vi "Set Frame Position (Time).vi"(8 "error in (no error)":errorcluster, 10 "Time (ms)":u64, 11 "Reader in":refnum<class "Reader.lvclass">) -> (0 "error out":errorcluster, 3 "Reader":refnum<class "Reader.lvclass">)   [LabVIEW 2020, in "video_io.lvlib" / "Reader.lvclass"]
uses:
  Reader.lvclass
  Reader.lvclass/Reader.ctl
  acb2feee-aaa4-4f40-955f-c8ac8e9dff35.vi
  <vilib>/Utility/error.llb/Error Cluster From Error Code.vi
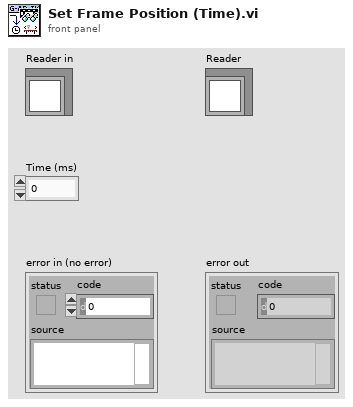
[diagram p1: front panel]
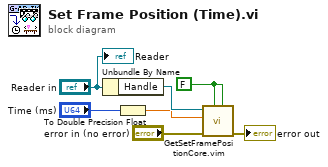
[diagram p0: block diagram]
diagram:
  w1 = FALSE ("Get")
  n1 = Unbundle By Name("Reader in") -> ("Handle"=w7:refnum<data-value>)
  n2 = To Double Precision Float(number="Time (ms)") -> (double precision float=w3:dbl)
  n3 = call "GetSetFramePositionCore.vim"("As Frame Index"=w1, "Get"=w1, "error in (no error)"="error in (no error)", "Position In"=w3, "Handle"=w7) -> ("error out"=→"error out":errorcluster)  [unwired: 5 in, 1 out]
  "Reader" <- "Reader in"
